vi "GT Get Watch Address.vi"(6 "count":i16, 7 "pAddress":u32, 8 "error in (no error)":errorcluster caption="错误输入（无错误）", 9 "index":i16, 10 "type":i16, 11 "cardNum":i16) -> (0 "error out":errorcluster caption="错误输出", 3 "function return":i16, 5 "pAddress out":u32)   [LabVIEW 2020, in "gts1.lvlib"]
doc: "GT_API GT_GetWatchAddress(short cardNum,short type,short index,unsigned long *pAddress,short count=1);"
uses:
  gts1.lvlib
  dll/32bit/multi_card/gts.dll
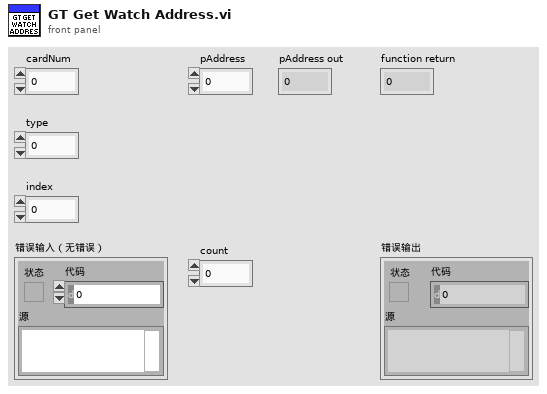
[diagram p1: front panel]
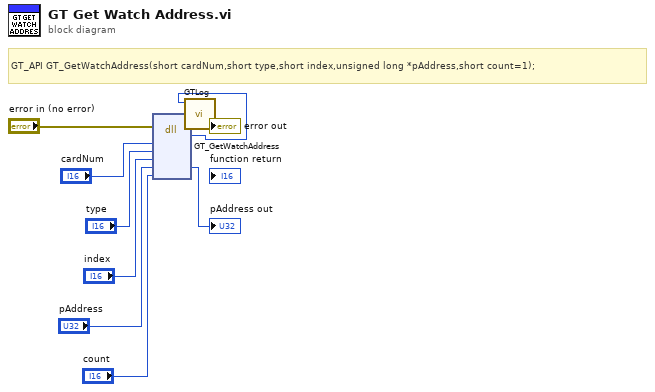
[diagram p0: block diagram]
diagram:
  # "GT_API GT_GetWatchAddress(short cardNum,short type,short index,unsigned long *pAddress,short count=1);"
  n1 = dll-call lib="C:/1228/dll/32bit/multi_card/gts.dll" fn="GT_GetWatchAddress"(error in="error in (no error)", "cardNum"="cardNum", "type"="type", "index"="index", "pAddress"="pAddress", "count"="count") -> (error out=w3:errorcluster, w1:i16, "pAddress"=→"pAddress out":u32)  [unwired: 6 in, 1 out]
  n2 = call "GTLog.vi"("error in (no error)"=w3, "Numeric"=w1) -> ("error out"=→"error out":errorcluster)  [unwired: 9 in]
